vi "Validate.vi"(8 "error in (no error)":errorcluster, 10 "Mock.lvclass":refnum<class "Mock.lvclass">, 11 "LUnit Test Case In":refnum<class "Test Case.lvclass">) -> (0 "error out":errorcluster, 3 "LUnit Test Case Out":refnum<class "Test Case.lvclass">)   [LabVIEW 2020, in "Mock.lvclass"]
uses:
  Mock.lvclass
  <vilib>/Astemes/LUnit/Test Case.lvclass
  Mock.lvclass/Mock.ctl
  <vilib>/Astemes/LUnit/Test Case.lvclass/Test Case.ctl
  <vilib>/Astemes/LUnit/Append Fail Result.vi
  <vilib>/Astemes/LUnit/Append Pass Result.vi
  Expectation/Expectation.lvclass
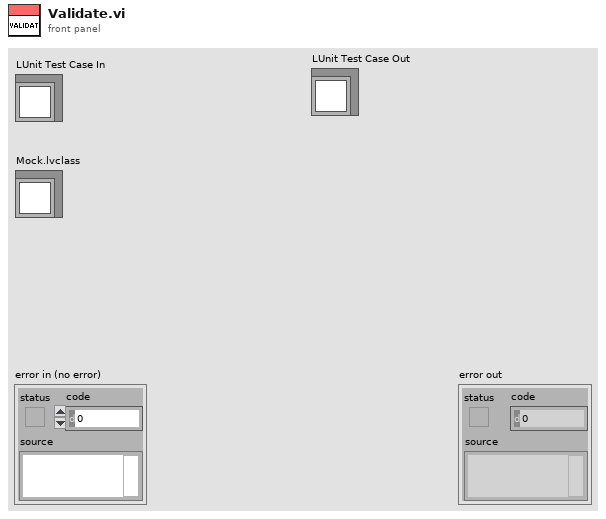
[diagram p1: front panel]
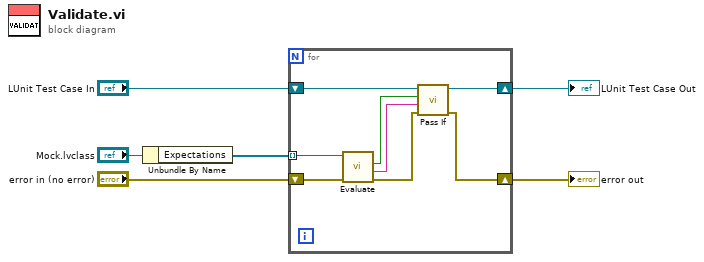
[diagram p0: block diagram]
diagram:
  n1 = Unbundle By Name("Mock.lvclass") -> ("Expectations"=w1:refnum<class "Expectation.lvclass">[])
  n2 = for {
    shift-right: [w13] -> w5
    shift-left: "LUnit Test Case In" -> [w14]
    shift-right: [w12] -> w3
    shift-left: "error in (no error)" -> [w11]
    tunnel: w1 -> [w9] mode=indexing
    n3 = call-dynamic "Evaluate.vi"("error in (no error)"=w11, "Expectation in"=w9) -> ("error out"=w10:errorcluster, "Message"=w7:string, "Passed?"=w8:bool)  [unwired: 7 in]
    n4 = call <vilib>:"Pass If.vi"("error in (no error)"=w10, "Message"=w7, "Pass?"=w8, "LUnit Test Case In"=w14) -> ("error out"=w12:errorcluster, "LUnit Test Case Out"=w13:refnum<class "Test Case.lvclass">)  [unwired: 6 in]
  }
  "error out" <- w3
  "LUnit Test Case Out" <- w5
